vi "TEST_L0_MAJ_(3RD)_NEW.vi"(7 "Serial Number":string="testFile", 8 "error in":errorcluster, 11 "Instrument VISA in":T1={"AWG VISA"="generadorpulsos", "Oscilloscope  VISA "="Oscilloscope", "Integration Board IP"="172.16.7.43", "connection ID"=refnum, "report out"=refnum, "report file path"=path "C:/Documents and Settings/CTA_LAB01/Desktop/L0_Asic/L0 Asic Test Data"}) -> (0 "error out":errorcluster, 3 "Instrument VISA out":T1={"AWG VISA"="generadorpulsos", "Oscilloscope  VISA "="Oscilloscope", "Integration Board IP"="172.16.7.43", "connection ID"=refnum, "report out"=refnum, "report file path"=path "C:/Documents and Settings/CTA_LAB01/Desktop/L0_Asic/L0 Asic Test Data"}, 5 "ThresholdOut":i32[][](array[numeric])=[[400, 400, 400, 400, 400, 400, 520], [400, 400, 400, 400, 400, 400, 520], [400, 400, 400, 400, 400, 400, 480], [400, 400, 400, 400, 400, 400, 400], [400, 400, 400, 400, 400, 400, 400]])   [LabVIEW 2009]
uses:
  <vilib>/Utility/NIReport.llb/NI_report.lvclass
  <vilib>/Utility/NIReport.llb/HTML/NI_HTML.lvclass
  Sum_Abrilader/L0_Sum_Adder Folder/C/Program Files/National Instruments/LabVIEW 2012/instr.lib/Agilent 8000 Series/Public/Configure/Configure Math (Binary Operation).vi
  <instrlib>/Agilent 8000 Series/Public/Data/Low Level/Fetch Measurement (More).vi
  <instrlib>/Agilent 8000 Series/Agilent 8000 Series.lvlib
panel:
  in  "Threshold Limits":i32[](array[numeric])=[300, 1024]
  in  "Voltages comprobation":dbl[](array[numeric])=[0.05, 0.1, 0.2, 0.5, 0.8]
  in  "Channels":i32[](array[numeric])=[0, 1, 2, 3, 4, 5, 6]
  out "threshold out":i32=400
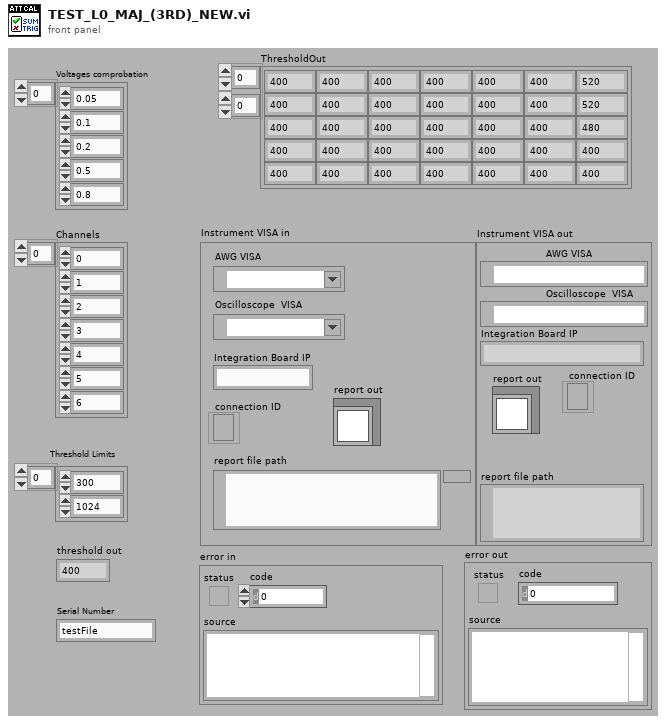
[diagram p1: front panel]
types:
  T1 = cluster{"AWG VISA":refnum<visa-resource-name>, "Oscilloscope  VISA ":refnum<visa-resource-name>, "Integration Board IP":string, "connection ID":refnum<k5>, "report out":refnum<class "NI_report.lvclass">, "report file path":path}
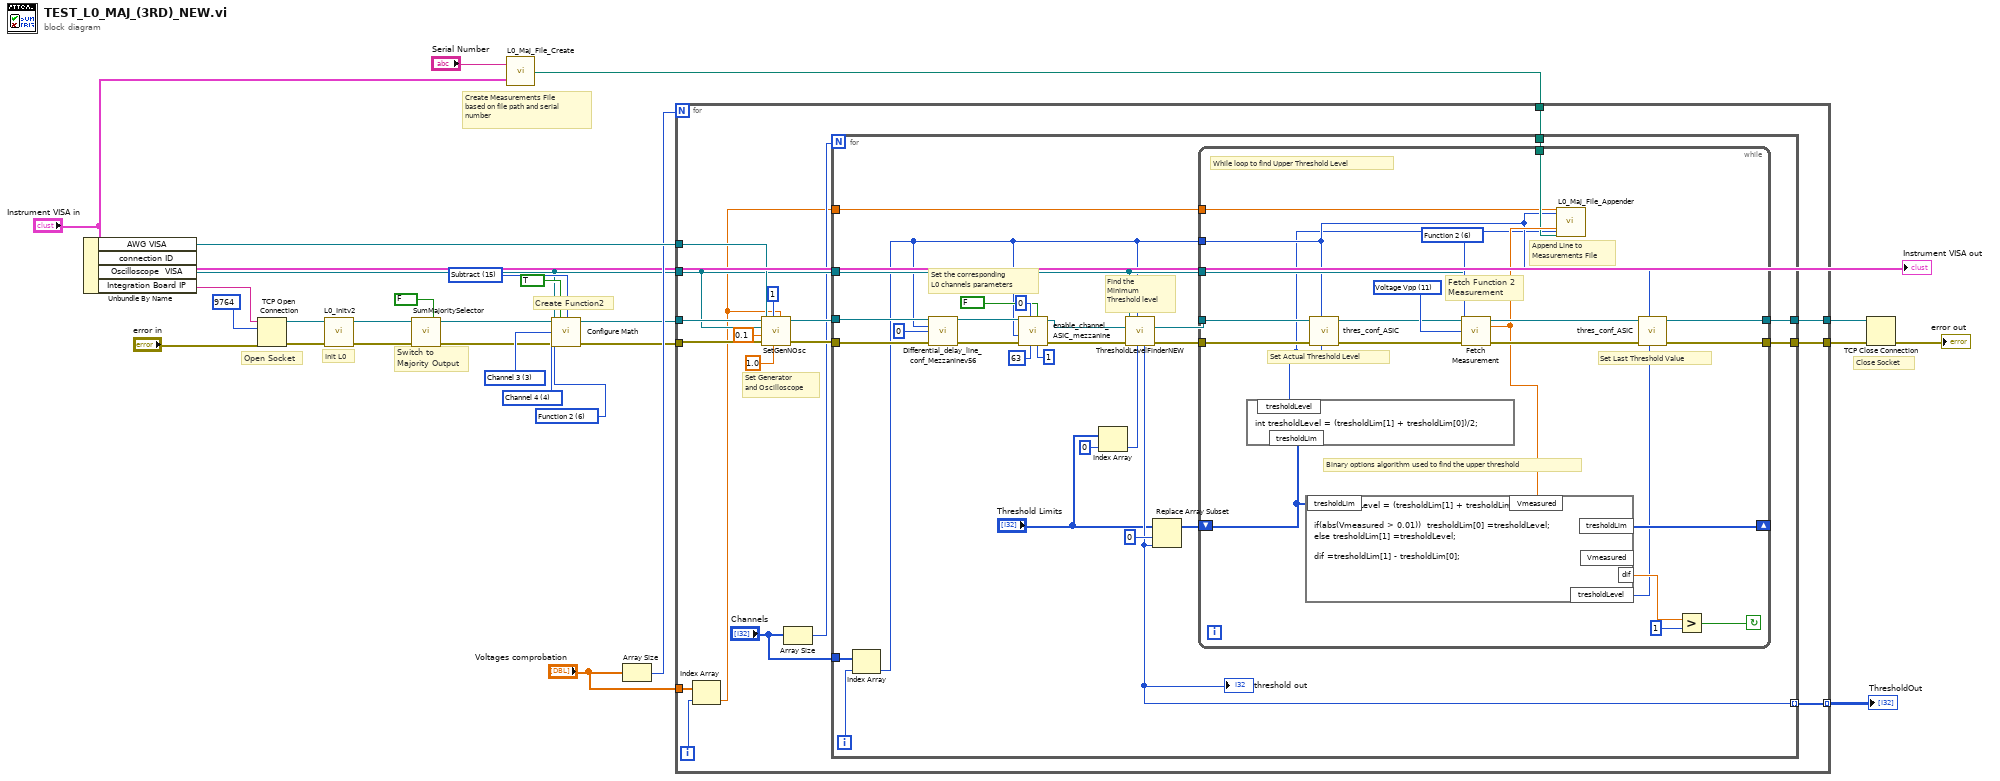
[diagram p0: block diagram]
diagram:
  w7 = u16 6 items=["Function 1"=5, "Function 2"=6, "Function 3"=7, "Function 4"=8] ("Math Channel (5: Function 1)")
  w8 = u16 15 items=["Add"=12, "Divide"=13, "Multiply"=14, "Subtract"=15, "Common Mode"=16, "Versus"=17] ("Math Operation (12: Add)")
  w6 = 3 items=["Channel 1"=1, "Channel 2"=2, "Channel 3"=3, "Channel 4"=4] ("Channel (1: Channel 1)")
  w5 = 4 items=["Channel 1"=1, "Channel 2"=2, "Channel 3"=3, "Channel 4"=4] ("Channel (1: Channel 1)")
  # "Close Socket"
  # "Create Function2"
  # "Switch to \nMajority Output"
  # "Init L0"
  # "Open Socket"
  # "Create Measurements File\nbased on file path and serial\nnumber"
  n1 = Unbundle By Name("Instrument VISA in") -> ("AWG VISA"=w17:refnum<visa-resource-name>, "Oscilloscope  VISA"=w1:refnum<visa-resource-name>, "Integration Board IP"=w23:string)  [unwired: 1 out]
  n2 = TCP Open Connection(address=w23, remote port or service name=u16 9764, error in (no error)="error in") -> (connection ID=w22:refnum<k5>, error out=w21:errorcluster)  [unwired: 2 in]
  n3 = call "L0_Initv2.vi"("error in"=w21, "connection ID in"=w22) -> ("error out"=w20:errorcluster, "connection ID out"=w19:refnum<k5>)  [unwired: 8 in]
  n4 = call "SumMajoritySelector.vi"("On Sum\nOff Majority"=FALSE ("On Sum\nOff Majority"), "error in (no error)"=w20, "connection ID"=w19) -> ("error out"=w3:errorcluster, "connection ID out"=w4:refnum<k5>)  [unwired: 5 in]
  n5 = call "L0_Maj_File_Create.vi"("input cluster"="Instrument VISA in", "Serial Number"="Serial Number") -> ("appended path"=w10:path)
  n6 = call-poly "Configure Math.vi"("VISA resource name"=w1, "Enable Math Channel (T:Enable)"=TRUE, "Math Operation (12: Add)"=w8, "Math Channel (5: Function 1)"=w7, "Math Operand (1: Channel 1)"=w6, "Math Operand (2: Channel 2)"=w5, "error in (no error)"=w3) -> ("error out"=w2:errorcluster)  [unwired: 7 in, 1 out]
  n7 = Array Size(array="Voltages comprobation") -> (size(s)=w15:i32)
  n8 = for {
    N: w15 -> [_]
    tunnel: [w44] -> w25
    tunnel: [w43] -> w24
    tunnel: w2 -> [w36]
    tunnel: w4 -> [w35]
    tunnel: w1 -> [w33]
    tunnel: w17 -> [w37]
    tunnel: "Voltages comprobation" -> [w42]
    tunnel: [w30] -> w13 mode=indexing
    tunnel: w10 -> [w29]
    i -> [w41]
    # "Set Generator\nand Oscilloscope"
    n9 = Index Array(array=w42, index=w41) -> (element=w28:dbl)
    n10 = call "SetGenNOsc.vi"("Input Voltage"=w28, "Amp Scaler"=1.0, "NChannels"=1, "error in (no error)"=w36, "Output Voltage"=0.1, "VISA resource name"=w33, "AWG VISA"=w37) -> ("error out 2"=w34:errorcluster)  [unwired: 4 in]
    n11 = Array Size(array="Channels") -> (size(s)=w32:i32)
    n12 = for {
      N: w32 -> [_]
      tunnel: [w57] -> w44
      tunnel: [w58] -> w43
      tunnel: w35 -> [w62]
      tunnel: w34 -> [w61]
      tunnel: w33 -> [w54]
      tunnel: "Channels" -> [w60]
      tunnel: [w51] -> w30 mode=indexing
      tunnel: w29 -> [w49]
      tunnel: w28 -> [w48]
      i -> [w59]
      # "Find the\nMinimum \nThreshold level"
      # "Set the corresponding\nL0 channels parameters"
      n13 = Index Array(array=w60, index=w59) -> (element=w53:i32)
      n14 = call "Differential_delay_line_conf_Mezzaninev56.vi"("connection ID"=w62, "channel"=w53, "Delay value"=u16 0, "error in (no error)"=w61) -> ("connection ID out"=w69:refnum<k5>, "error out 2"=w70:errorcluster)  [unwired: 4 in, 6 out]
      n15 = call "enable_channel_ASIC_mezzanine.vi"("Clip_sel_b"=u32 1, "maj/sum"=FALSE, "Ib_clipVb"=u32 63, "Att gain"=u32 0, "error in"=w70, "Channel"=w53, "connection ID"=w69) -> ("error out"=w63:errorcluster, "connection ID out"=w64:refnum<k5>)  [unwired: 2 in, 1 out]
      n16 = Index Array(array="Threshold Limits", index=0) -> (element=w45:i32)
      n17 = call "ThresholdLevelFinderNEW.vi"("Initial Threshold"=w45, "Channel"=w53, "error in (no error)"=w63, "connection ID"=w64, "VISA resource name"=w54) -> ("error out"=w56:errorcluster, "connection ID out"=w55:refnum<k5>, "threshold out"=w51:i32)  [unwired: 2 in, 2 out]
      "threshold out" <- w51
      n18 = Replace Array Subset(array="Threshold Limits", new element=w51, index=u32 0 ("Att gain")) -> (w50:i32[])
      n19 = while {
        tunnel: [w92] -> w58
        tunnel: [w91] -> w57
        tunnel: w56 -> [w90]
        tunnel: w55 -> [w89]
        tunnel: w54 -> [w86]
        tunnel: w53 -> [w73]
        shift-right: [w78] -> _
        shift-left: w50 -> [w77]
        tunnel: w49 -> [w75]
        tunnel: w48 -> [w74]
        stop <- w81 continue-if-true
        w88 = 11 items=["Rise Time", "Fall Time", "Frequency", "Period", "Voltage RMS(AC)", "Voltage RMS(DC)", "Voltage RMS (AC,cycle)", "Voltage RMS (DC,cycle)", "Voltage Max", "Voltage Min", "Voltage Middle", "Voltage Vpp", "Voltage High", "Voltage Low", "Voltage Average", "Voltage Average (cycle)", "Width Negative", "Width Positive", "Duty Cycle Positive", "Amplitude", "Overshoot", "Preshoot", "Voltage Base", "Voltage Upper", "Time Max", "Time Min", "Color Grade Crossing", "Color Grade Eye Width", "Color Grade Eye Height", "Color Grade Eye Q-Factory", "Color Grade Eye Duty Cycle Distortion(Percent)", "Color Grade Eye Duty Cycle Distortion(Time)", "Color Grade Eye Jitter(PP)", "Color Grade Eye Width(RMS)", "Cycle-cycle Duty Jitter(Rising)", "Cycle-cycle Duty Jitter(Falling)", "Cycle-cycle Jitter(Rising)", "Cycle-cycle Jitter(Falling)", "Cycle-cycle - Width", "Cycle-cycle + Width", "Date Rate", "Unit Interval", "FFT Delta Frequency", "FFT Delta Magnitude", "FFT Frequency", "FFT Magnitude", "Slew Rate", "Area (Entire Display)", "Area(Single Cycle)", "Duty Cycle (Rising)", "Duty Cycle (Falling)"] ("Measurement Function (0: Rise Time)")
        w87 = 6 items=["Channel 1"=1, "Channel 2"=2, "Channel 3"=3, "Channel 4"=4, "Function 1"=5, "Function 2"=6, "Function 3"=7, "Function 4"=8, "Memory 1"=9, "Memory 2"=10, "Memory 3"=11, "Memory 4"=12] ("Channel (1: Channel 1)")
        # "Binary options algorithm used to find the upper threshold"
        # "Set Last Threshold Value"
        # "While loop to find Upper Threshold Level"
        # "Set Actual Threshold Level"
        # "Append Line to \nMeasurements File"
        # "Fetch Function 2\nMeasurement"
        n20 = formula code="int tresholdLevel = (tresholdLim[1] + tresholdLim[0])/2;"("tresholdLim"=w77) -> ("tresholdLevel"=w72:i32)
        n21 = call "thres_conf_ASIC.vi"("threshold"=w72, "Ring"=w73, "error out 3"=w90, "connection ID"=w89) -> ("error out 2"=w85:errorcluster, "connection ID out"=w83:refnum<k5>)  [unwired: 4 in, 2 out]
        n22 = call-poly <instrlib>:"Fetch Measurement.vi"("VISA resource name"=w86, "Channel (1: Channel 1)"=w87, "Measurement Function (0: Rise Time)"=w88, "error in (no error)"=w85) -> ("Measurement"=w79:dbl, "error out"=w84:errorcluster)  [unwired: 9 in, 1 out]
        n23 = formula code="int tresholdLevel = (tresholdLim[1] + tresholdLim[0])/2;\n\nif(abs(Vmeasured > 0.01))  tresholdLim[0] =tresholdLevel;\nelse tresholdLim[1] =tresholdLevel;\n\ndif =tresholdLim[1] - tresholdLim[0];"("Vmeasured"=w79, "tresholdLim"=w77) -> ("dif"=w80:dbl, "tresholdLevel"=w76:i32, "tresholdLim"=w78:i32[])  [unwired: 1 out]
        n24 = call "L0_Maj_File_Appender.vi"("Vin"=w74, "CH"=w73, "Vmeas"=w79, "Threshold"=w72, "file path (dialog if empty)"=w75) -> ()  [unwired: 23 in]
        n25 = call "thres_conf_ASIC.vi"("threshold"=w76, "Ring"=w73, "error out 3"=w84, "connection ID"=w83) -> ("error out 2"=w91:errorcluster, "connection ID out"=w92:refnum<k5>)  [unwired: 4 in, 2 out]
        n26 = Greater?(x=w80, y=1) -> (0:w81:bool)
      }
    }
  }
  "ThresholdOut" <- w13
  n27 = TCP Close Connection(connection ID=w24, error in (no error)=w25) -> (error out=→"error out":errorcluster)  [unwired: 1 in, 1 out]
  "Instrument VISA out" <- "Instrument VISA in"
